vi "setUp.vi"(8 "error in (no error)":errorcluster, 11 "reference in":refnum<class "FPGA Addon Test Class.lvclass">) -> (0 "error out":errorcluster, 3 "reference out":refnum<class "FPGA Addon Test Class.lvclass">)   [LabVIEW 2019]
doc: "setUp runs prior to the test method during test execution. Use this method to initialize any object data required by your tests."
uses:
  FPGA Addon Test Class.lvclass
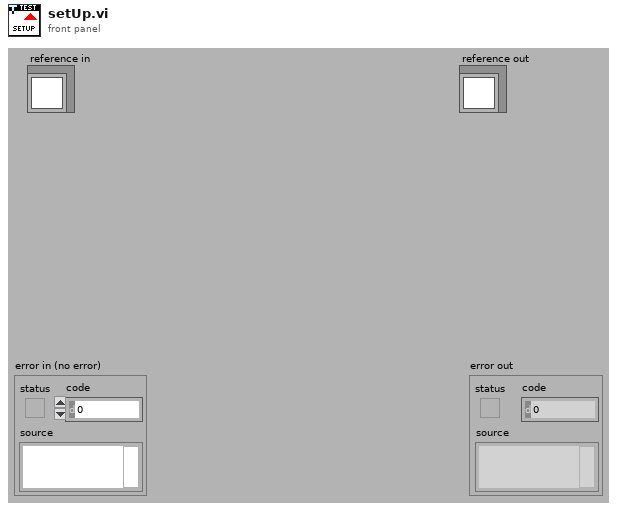
[diagram p1: front panel]
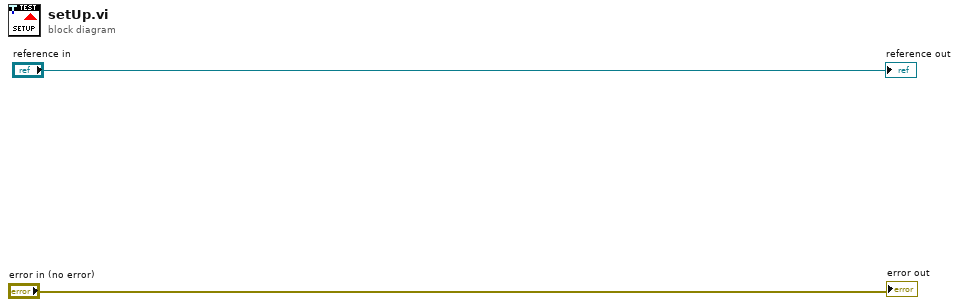
[diagram p0: block diagram]
diagram:
  "error out" <- "error in (no error)"
  "reference out" <- "reference in"
